vi "Close File.vi"(8 "error in":errorcluster, 11 "CSV in":refnum<class "CSV.lvclass">) -> (0 "error out":errorcluster, 3 "CSV out":refnum<class "CSV.lvclass">)   [LabVIEW 2019, in "ManejoArchivos.lvlib" / "CSV.lvclass"]
uses:
  CSV.lvclass
  CSV.lvclass/CSV.ctl
  Read file Ref.vi
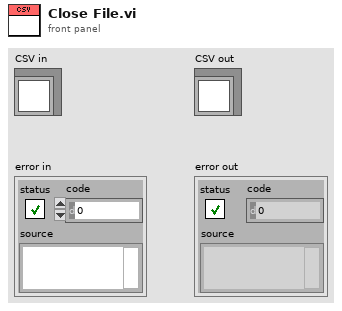
[diagram p1: front panel]
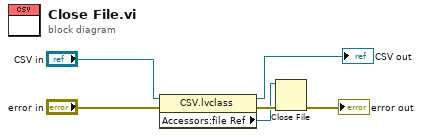
[diagram p0: block diagram]
diagram:
  n1 = property class="CSV.lvclass"(reference="CSV in", error in="error in") -> (reference out=→"CSV out":refnum<class "CSV.lvclass">, error out=w5:errorcluster, "Accessors:file Ref"=w1:refnum<file>)
  n2 = Close File(refnum=w1, error in=w5) -> (error out=→"error out":errorcluster)  [unwired: 1 out]
